vi "exercicio 1.vi"() -> ()   [LabVIEW 2025]
panel:
  out "Slide":u8(slide) scale=0.0..200.0
  in  "Numeric":dbl
  in  "Array 2-1":dbl
  in  "Array 2-0":dbl
  in  "Array 1-0":dbl
  in  "Array 1-1":dbl
  out "i value":i32
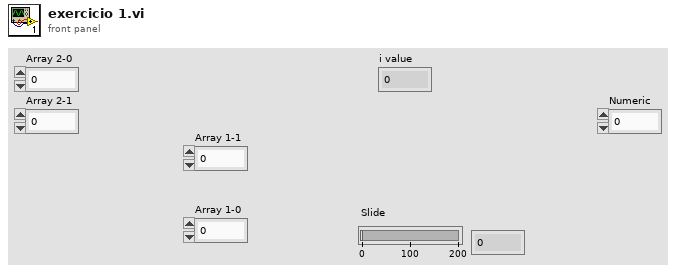
[diagram p1: front panel]
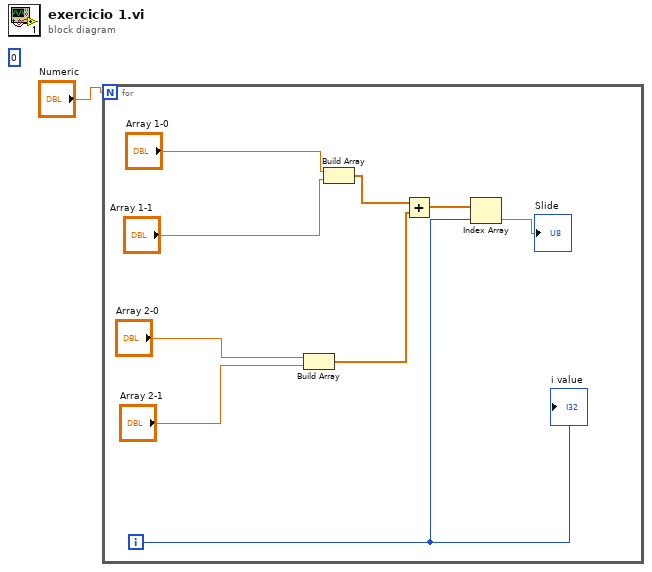
[diagram p0: block diagram]
diagram:
  (unwired) 0
  n1 = for {
    N: "Numeric" -> [_]
    i -> [w4]
    n2 = Build Array("Array 2-0", "Array 2-1") -> (w6:dbl[])
    n3 = Build Array("Array 1-0", "Array 1-1") -> (w9:dbl[])
    n4 = Add(x=w9, y=w6) -> (x+y=w5:dbl[])
    n5 = Index Array(array=w5, index=w4) -> (element=→"Slide":dbl)
    "i value" <- w4
  }
